vi "Destroy Parallel Events.vi"(8 "error in (no error)":errorcluster, 11 "CIFPluginManager in":refnum<class "CIFPluginManager.lvclass">) -> (0 "error out":errorcluster, 3 "CIFPluginManager out":refnum<class "CIFPluginManager.lvclass">)   [LabVIEW 2021, in "CIFPluginManager.lvclass"]
uses:
  CIFPluginManager.lvclass
  CIFPluginManager.lvclass/CIFPluginManager.ctl
  typedef/Parallel Events.ctl
  typedef/Loader Load Command.ctl
  typedef/Loader Type.ctl
  typedef/Plugin Load Command.ctl
  typedef/Discover Command.ctl
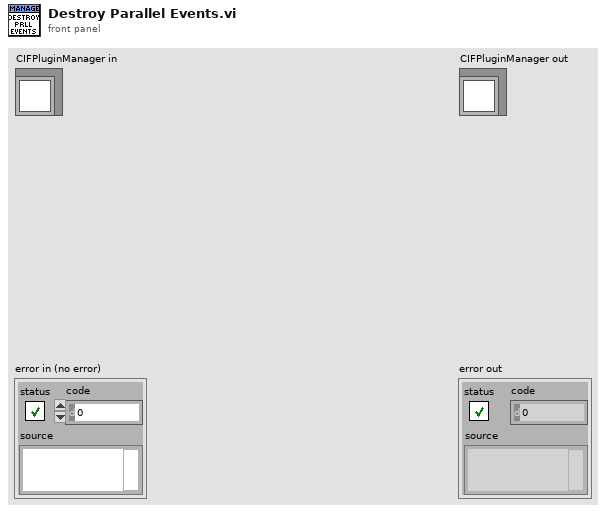
[diagram p1: front panel]
types:
  T1 = typedef "CIFPluginManager.lvclass/Parallel Events.ctl" = cluster{"Shutdown":refnum<user-event>, "Load Loader Events":refnum<user-event>, "Load Plugin Events":refnum<user-event>, "Trigger Discovery":refnum<user-event>, "Discover Events":refnum<user-event>}
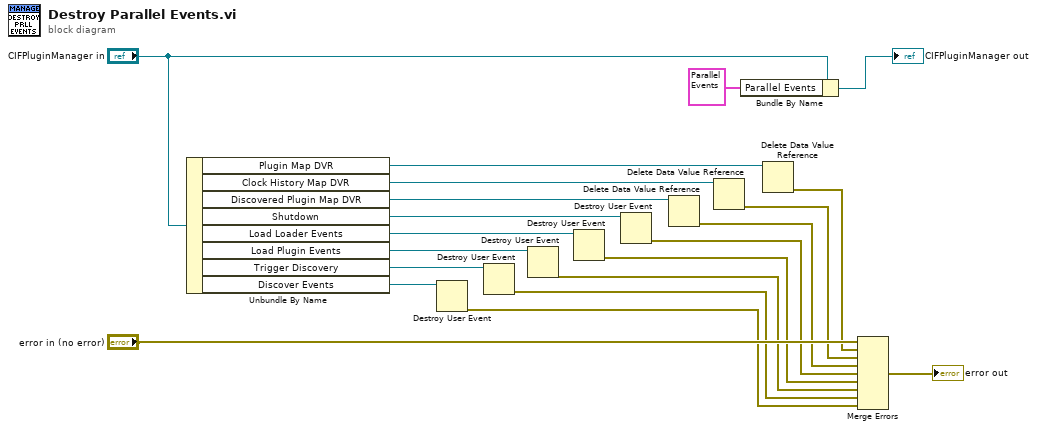
[diagram p0: block diagram]
diagram:
  n1 = Unbundle By Name("CIFPluginManager in") -> ("Plugin Map DVR"=w12:refnum<data-value>, "Clock History Map DVR"=w13:refnum<data-value>, "Discovered Plugin Map DVR"=w14:refnum<data-value>, "Shutdown"=w17:refnum<user-event>, "Load Loader Events"=w18:refnum<user-event>, "Load Plugin Events"=w6:refnum<user-event>, "Trigger Discovery"=w5:refnum<user-event>, "Discover Events"=w2:refnum<user-event>)
  n2 = Destroy User Event(user event=w2) -> (error out=w1:errorcluster)  [unwired: 1 in]
  n3 = Destroy User Event(user event=w5) -> (error out=w3:errorcluster)  [unwired: 1 in]
  n4 = Destroy User Event(user event=w6) -> (error out=w4:errorcluster)  [unwired: 1 in]
  n5 = Destroy User Event(user event=w18) -> (error out=w7:errorcluster)  [unwired: 1 in]
  n6 = Destroy User Event(user event=w17) -> (error out=w8:errorcluster)  [unwired: 1 in]
  n7 = Delete Data Value Reference(data value reference=w14) -> (error out=w9:errorcluster)  [unwired: 1 in, 1 out]
  n8 = Delete Data Value Reference(data value reference=w13) -> (error out=w10:errorcluster)  [unwired: 1 in, 1 out]
  n9 = Bundle By Name(cluster="CIFPluginManager in", "Parallel Events"=T1 {"Shutdown"=refnum, "Load Loader Events"=refnum, "Load Plugin Events"=refnum, "Trigger Discovery"=refnum, "Discover Events"=refnum} ("Discovery Events")) -> (→"CIFPluginManager out":refnum<class "CIFPluginManager.lvclass">)
  n10 = Delete Data Value Reference(data value reference=w12) -> (error out=w11:errorcluster)  [unwired: 1 in, 1 out]
  n11 = Merge Errors("error in (no error)", w11, w10, w9, w8, w7, w4, w3, w1) -> (→"error out":errorcluster)
